vi "File.Create Filesafe TimeStamp.vi"(7 "Start Time":timestamp, 10 "Suffix":string="ABC123", 11 "Prefix":string="ABC123") -> (3 "FileFriendly Text with Timestamp":string)   [LabVIEW 2024]
uses:
  File Utils.lvlib
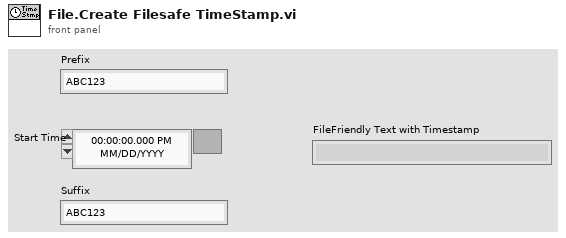
[diagram p1: front panel]
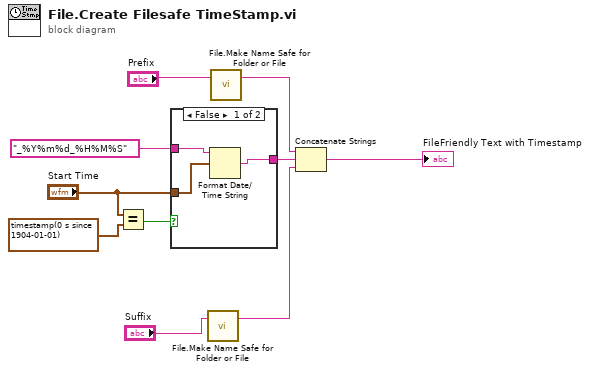
[diagram p0: block diagram]
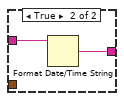
[diagram p2: hidden frame]
diagram:
  n1 = Equal?(x="Start Time", y=timestamp(0 s since 1904-01-01) ("Start Time")) -> (x = y?=w2:bool)
  n2 = case shown="False" w2 {
    tunnel: "_%Y%m%d_%H%M%S" ("time format string (%c)") -> [w13 w15]
    tunnel: [w11 w14] -> w9
    tunnel: "Start Time" -> [w12 _]
    frame False {
      n3 = Format Date/Time String(time format string (%c)=w13, seconds (now)=w12) -> (date/time string=w11:string)  [unwired: 1 in]
    }
    frame True {
      n4 = Format Date/Time String(time format string (%c)=w15) -> (date/time string=w14:string)  [unwired: 2 in]
    }
  }
  n5 = call "File.Make Name Safe for Folder or File.vi"("File Name"="Suffix") -> ("Fixed Name"=w4:string)  [unwired: 2 in]
  n6 = call "File.Make Name Safe for Folder or File.vi"("File Name"="Prefix") -> ("Fixed Name"=w6:string)  [unwired: 2 in]
  n7 = Concatenate Strings(w6, w9, w4) -> (→"FileFriendly Text with Timestamp":string)
